vi "Load Display Settings.vi"(8 "error in (no error)":errorcluster, 11 "HIJ IMAQdx Display in":refnum<class "HIJ IMAQdx Display.lvclass">) -> (0 "error out":errorcluster, 3 "HIJ IMAQdx Display out":refnum<class "HIJ IMAQdx Display.lvclass">)   [LabVIEW 2014, in "HIJ IMAQdx Display.lvlib" / "HIJ IMAQdx Display.lvclass"]
doc: "Lade Anzeigeeinstellungen. Typischer Weise sind sie von der Kamera abhängig. Also wird aus dem Konfigpfad die Datei <Camera name>.xdcnf geladen."
uses:
  HIJ IMAQdx Display.lvclass
  HIJ Vision Display/HIJ Vision Display/Named ROI.ctl
  HIJ Vision Display/HIJ Vision Display/DisplaySettings.ctl
  HIJ Vision Display/HIJ Vision Display/HIJ Vision Display.lvclass/HIJ Vision Display.ctl
  HIJ IMAQdx Display.lvclass/HIJ IMAQdx Display.ctl
  HIJ Vision Display/HIJ Vision Display/Write Display settings.vi
  HIJ Vision Display/HIJ Vision Display/Write Saved ROIs.vi
  HIJ Vision Display/HIJ Vision Display/Write ROI 1.vi
  HIJ Vision Display/HIJ Vision Display/Read Display ref.vi
  Read ConfigDir.vi
  HIJ Vision Display/HIJ Vision Display/Read Image Source Name.vi
  HIJ Vision Display/HIJ Vision Display/HIJ Vision Display.lvclass
  Utility/POLARIS Vision utility.lvlib
panel:
  in  "ROI":T1 {"Contours"."Type" items=["No Selection", "Point", "Line", "Rectangle", "Oval", "Polygon", "Freehand Region", "Annulus", "Unused2", "Unused3", "Broken Line", "Freehand Line", "Rotated Rectangle"]}
  in  "Display settings":T2
  in  "Saved ROIs":T3[](array[typedef])
  in  "Image Center":cluster{"X":u32, "Y":u32}
  in  "Zoom":cluster{"X":i32, "Y":i32}
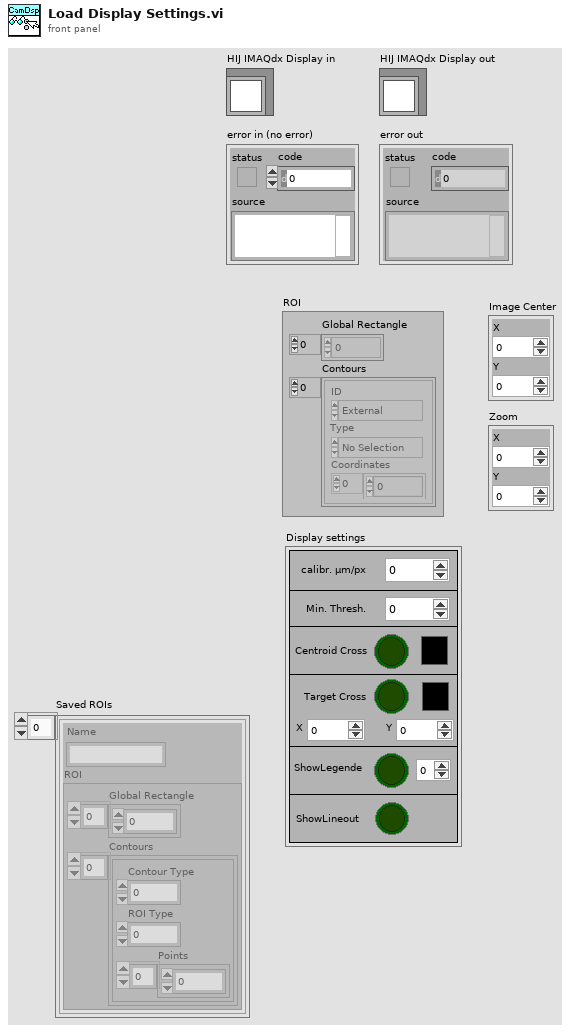
[diagram p1: front panel]
types:
  T1 = typedef "ROI Descriptor" = cluster{"Global Rectangle":i32[], "Contours":cluster{"ID":enum32{"External", "Internal"}, "Type":u32, "Coordinates":i32[]}[]}
  T2 = typedef "HIJ Vision Display.lvlib/HIJ Vision Display.lvclass/DisplaySettings.ctl" = cluster{"Min. Thresh.":sgl, "X":dbl, "Y":dbl, "ShowLineout":bool, "ScaleParts":i32, "ShowLegende":bool, "Target Cross":bool, "Centroid Cross":bool, "Target color":u32, "Centroid color":u32, "calibr. µm/px":sgl[unit]}
  T3 = typedef "HIJ Vision Display.lvlib/HIJ Vision Display.lvclass/Named ROI.ctl" = cluster{"ROI":cluster{"Global Rectangle":i32[], "Contours":cluster{"Contour Type":u32, "ROI Type":u32, "Points":i32[]}[]}, "Name":string}
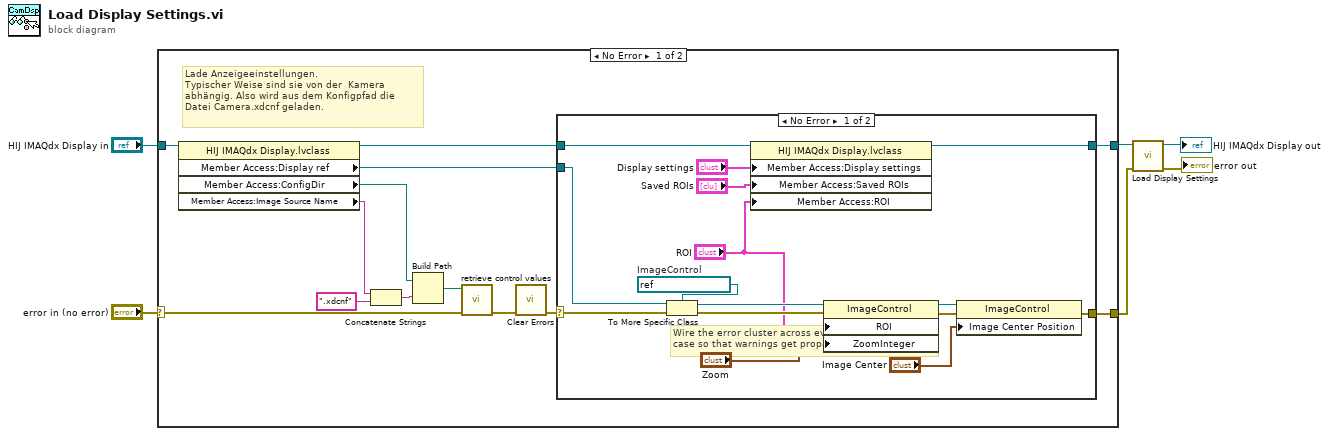
[diagram p0: block diagram]
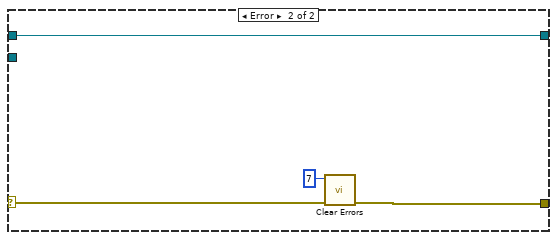
[diagram p2: hidden frame]
diagram:
  n1 = case shown="No Error" "error in (no error)" {
    selector: "error in (no error)" -> [w13 w40]
    tunnel: [w10 w40] -> w2
    tunnel: [w14 w39] -> w4
    tunnel: "HIJ IMAQdx Display in" -> [w9 w39]
    frame No Error {
      # "Lade Anzeigeeinstellungen.\nTypischer Weise sind sie von der  Kamera\nabhängig. Also wird aus dem Konfigpfad die \nDatei Camera.xdcnf geladen."
      # "Wire the error cluster across even in the \"No Error\"\ncase so that warnings get propagated."
      n2 = property class="HIJ IMAQdx Display.lvclass"(reference=w9) -> (reference out=w12:refnum<class "HIJ IMAQdx Display.lvclass">, "Member Access:Display ref"=w11:refnum<vi>, "Member Access:ConfigDir"=w7:path, "Member Access:Image Source Name"=w8:string)  [unwired: 1 in, 1 out]
      n3 = Concatenate Strings(w8, ".xdcnf" ("string")) -> (w17:string)
      n4 = Build Path(base path=w7, name or relative path=w17) -> (appended path=w15:path)
      n5 = call "retrieve control values.vi"("error in (no error)"=w13, "path"=w15) -> ("error out"=w16:errorcluster)  [unwired: 8 in, 1 out]
      n6 = call <vilib>:"Clear Errors.vi"("error in (no error)"=w16) -> ("error out"=w19:errorcluster)  [unwired: 5 in, 1 out]
      n7 = case shown="No Error" w19 {
        selector: w19 -> [w32 w38]
        tunnel: [w21 w36] -> w10
        tunnel: [w24 w37] -> w14
        tunnel: w12 -> [w25 w37]
        tunnel: w11 -> [w30 _]
        frame No Error {
          w29 = refnum<vi> refnum  # ImageControl
          n8 = To More Specific Class(target class=w29, reference=w30, error in=w32) -> (specific class reference=w33:refnum<vi>, error out=w34:errorcluster)
          n9 = property class="HIJ IMAQdx Display.lvclass"(reference=w25, "Member Access:Display settings"="Display settings", "Member Access:Saved ROIs"="Saved ROIs", "Member Access:ROI"="ROI") -> (reference out=w24:refnum<class "HIJ IMAQdx Display.lvclass">)  [unwired: 1 in, 1 out]
          n10 = property class="ImageControl"(reference=w33, error in=w34, "ROI"="ROI", "ZoomInteger"="Zoom") -> (reference out=w26:refnum<vi>, error out=w27:errorcluster)
          n11 = property class="ImageControl"(reference=w26, error in=w27, "Image Center Position"="Image Center") -> (error out=w21:errorcluster)  [unwired: 1 out]
        }
        frame Error {
          n12 = call <vilib>:"Clear Errors.vi"("error in (no error)"=w38, "specific error code to clear (0: all)"=7) -> ("error out"=w36:errorcluster)  [unwired: 4 in, 1 out]
        }
      }
    }
    frame Error {
    }
  }
  n13 = call-parent "Load Display Settings.vi"("error in (no error)"=w2, "AF IMAQ Display in"=w4) -> ("error out"=→"error out":errorcluster, "AF IMAQ Display out"=→"HIJ IMAQdx Display out":refnum<class "HIJ IMAQdx Display.lvclass">)  [unwired: 8 in]
